vi "RunMeas.vi"(8 "error in (no error)":errorcluster, 11 "ChromaAcLoad in":refnum<class "ChromaAcLoad.lvclass">) -> (0 "error out":errorcluster, 2 "variant":variant, 3 "ChromaAcLoad out":refnum<class "ChromaAcLoad.lvclass">)   [LabVIEW 2018, in "AcPwrPlugins.lvlib" / "ChromaAcLoad.lvclass"]
doc: "This VI (may) initiate the measurement and retrieves the measurement value from the device."
uses:
  ChromaAcLoad.lvclass
  AcPwrShared/clMeasurmentData.ctl
  AcPwrShared/clAcPwrAttributes.ctl
  <instrlib>/C63800/C63800.llb/C63800 M/F Overshoot Voltage.vi
  <instrlib>/C63800/C63800.llb/C63800 M/F Negative Peak Current.vi
  <instrlib>/C63800/C63800.llb/C63800 M/F Undershoot Voltage.vi
  <instrlib>/C63800/C63800.llb/C63800 M/F Apparent Power.vi
  <instrlib>/C63800/C63800.llb/C63800 M/F Power Reactive.vi
  <instrlib>/C63800/C63800.llb/C63800 M/F Power Factor.vi
  AcPwrShared/AcPwrShared.lvlib
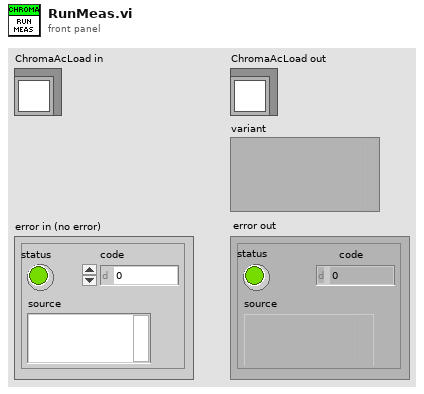
[diagram p1: front panel]
types:
  T1 = typedef "AcPwrPlugins.lvlib/ChromaAcLoad.lvclass/Device(s)Settings.ctl" = cluster{"Configuration Mode":enum16{"Constant Voltage (DC)", "Constant Power (DC)", "Constant Power (AC)", "Constant Current (DC)", "Constant Current (AC)", "Constant Resistance (DC)", "Constant Resistance (AC)", "Rectified Mode (DC)", "Inrush (AC)", "RLC CP (AC)", "RLC (AC)"}, "Phases":cluster{"Handle":string, "Name":string, "Phase Select":i32, "Instrument Options":string, "id query (T)":bool, "reset device (T)":bool, "Load Short Circuited":bool, "Line Synchronization":bool, "Load Current (A/Arms)":dbl, "Load Voltage (V/Vrms)":dbl, "Load Power (W)":dbl, "Load Resistance (Ohms)":dbl, "Load Current Peak Limit (A)":dbl, "Load Current Limit (A/Arms)":dbl, "Load Power Limit (W)":dbl, "Synch Frequency (Hz)":dbl, "Priority":enum16{"CF Only", "PF Only", "Both (CF)", "Both (PF)"}, "Crest Factor":dbl, "Power Factor":dbl, "Slew Rate":cluster{"Rise Slew Rate (A/ms)":i32, "Fall Slew Rate (A/ms)":i32}, "LC/RLC Mode":cluster{"Capacitance (uF)":i32, "Inductance (uH)":i32, "Series Resistance (Ohm)":dbl, "Parallel Resistance (Ohm)":dbl}, "Timing":cluster{"TimingOn":enum16{""}, "Hours":u32, "Minutes":u32, "Seconds":dbl, "CutoffVoltage":dbl}, "Connected":bool}[], "MeasName":string}
  T2 = typedef "AcPwrPlugins.lvlib/ChromaAcLoad.lvclass/Measurements.ctl" = cluster{"Handle":string, "Name":string, "Enabled":bool, "Measurement Value":dbl, "Hold Peak Current Measurement":bool, "btnMeasFetch":bool, "ProtectionStatusString":string, "Measurement Type":T3}[]
  T3 = typedef "AcPwrPlugins.lvlib/ChromaAcLoad.lvclass/MeasurementType.ctl" = enum16{"Voltage (Vrms or V)", "Current (Arms or A)", "Power (W)", "Peak Voltage (V)", "Peak Current (A)", "Peak Power (W)", "Frequency (Hz)", "Resistance (Ohms)", "Voltage Overshoot (V)", "Positive Peak Current (A)", "Voltage Undershoot (V)", "Negative Peak Current (A)", "Apparent Power (VA)", "Reacitive Power (VAR)", "Voltage THD", "Power Factor", "Current's Crest Factor"}
  T4 = typedef "AcPwrShared.lvlib/clMeasurmentData.ctl" = cluster{"MeasName":string, "XML Data":string, "WaveformData":waveform(dbl)[]}
  T5 = typedef "AcPwrShared.lvlib/clAcPwrAttributes.ctl" = cluster{"ProtectionStatusString":string, "Handle_MeasurementType":string, "Status Byte Register":cluster{"Busy":bool, "Remote Mode":bool, "Error in Queue":bool, "QUES=Questionable Status Summary":bool, "MAV = Message Available":bool, "ESB = Event Status Byte Summary":bool, "RQS = Request for Service":bool, "OPER = Operation Event Summary":bool}}
  T6 = cluster{"Handle":string, "Name":string, "Enabled":bool, "Measurement Value":dbl, "Hold Peak Current Measurement":bool, "btnMeasFetch":bool, "ProtectionStatusString":string, "Measurement Type":T3}
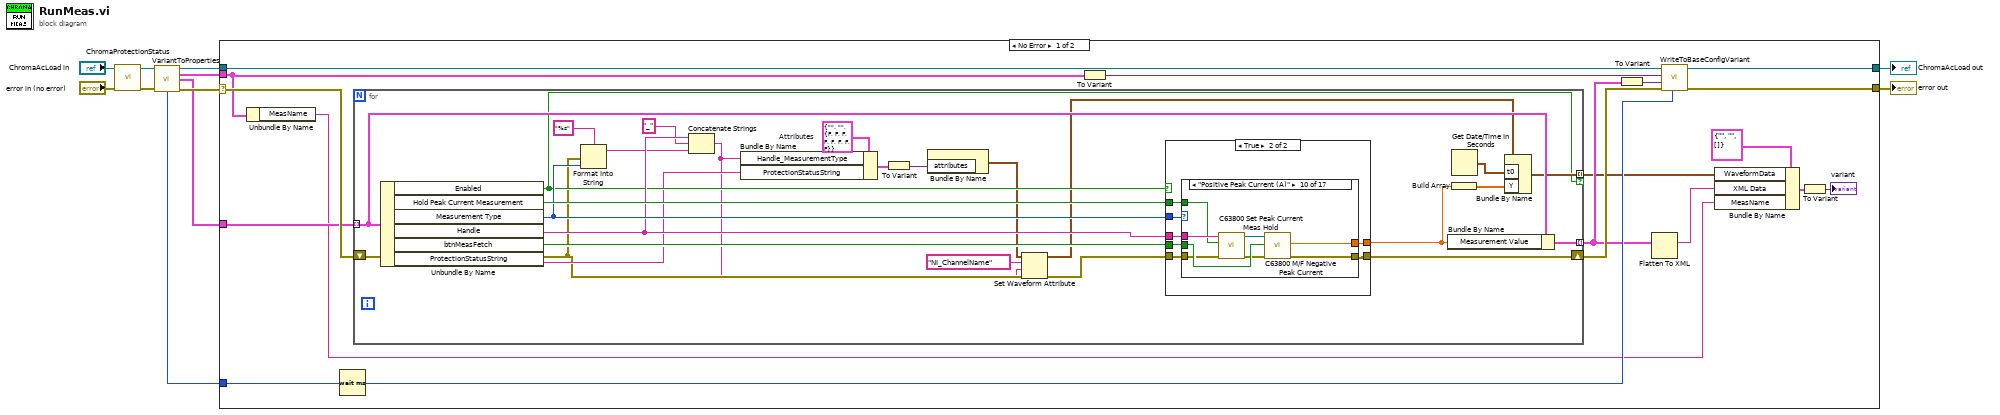
[diagram p0: block diagram]
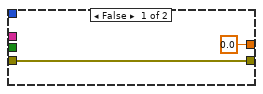
[diagram p2: hidden frame]
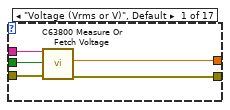
[diagram p3: hidden frame]
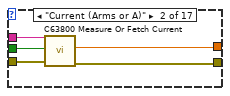
[diagram p4: hidden frame]
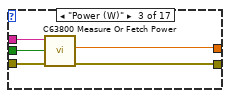
[diagram p5: hidden frame]
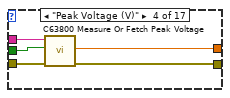
[diagram p6: hidden frame]
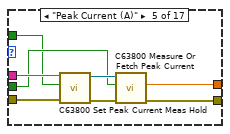
[diagram p7: hidden frame]
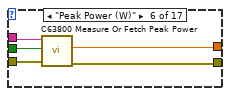
[diagram p8: hidden frame]
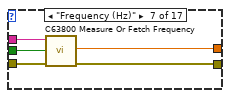
[diagram p9: hidden frame]
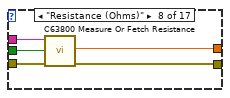
[diagram p10: hidden frame]
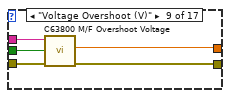
[diagram p11: hidden frame]
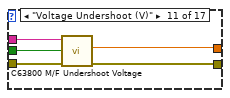
[diagram p12: hidden frame]
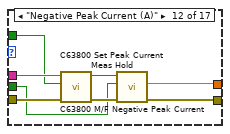
[diagram p13: hidden frame]
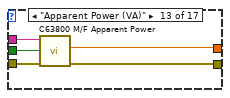
[diagram p14: hidden frame]
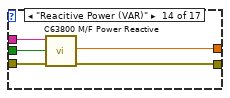
[diagram p15: hidden frame]
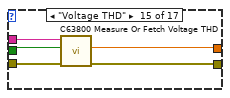
[diagram p16: hidden frame]
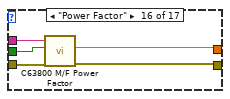
[diagram p17: hidden frame]
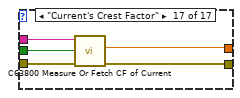
[diagram p18: hidden frame]
diagram:
  n1 = call "ChromaProtectionStatus.vi"("error in (no error)"="error in (no error)", "ChromaAcLoad in"="ChromaAcLoad in") -> ("error out"=w7:errorcluster, "ChromaAcLoad out"=w6:refnum<class "ChromaAcLoad.lvclass">)  [unwired: 8 in]
  n2 = call "VariantToProperties.vi"("ChromaAcLoad"=w6, "error in (no error)"=w7) -> ("ChromaAcLoad"=w5:refnum<class "ChromaAcLoad.lvclass">, "Device Properties"=w2:T1, "Meas"=w3:T2, "Measurement Refresh Time (ms)"=w1:u32, "error out"=w4:errorcluster)  [unwired: 7 in, 2 out]
  n3 = case shown="No Error" w4 {
    selector: w4 -> [w29 w158]
    tunnel: [w25 w159] -> w11
    tunnel: [w23 w158] -> w10
    tunnel: w5 -> [w27 w159]
    tunnel: w2 -> [w20 _]
    tunnel: w3 -> [w28 _]
    tunnel: w1 -> [w21 _]
    frame No Error {
      n4 = Unbundle By Name(w20) -> ("MeasName"=w12:string)
      n5 = Wait (ms)(milliseconds to wait=w21) -> (millisecond timer value=w18:u32)
      n6 = for {
        tunnel: w28 -> [w54] mode=indexing
        shift-right: [w52] -> w26
        shift-left: w29 -> [w32]
        tunnel: [w53] -> w17 mode=indexing
        tunnel: [w47] -> w14 mode=indexing if=w39
        w38 = T5 {"ProtectionStatusString"="", "Handle_MeasurementType"="", "Status Byte Register"={"Busy"=FALSE, "Remote Mode"=FALSE, "Error in Queue"=FALSE, "QUES=Questionable Status Summary"=FALSE, "MAV = Message Available"=FALSE, "ESB = Event Status Byte Summary"=FALSE, "RQS = Request for Service"=FALSE, "OPER = Operation Event Summary"=FALSE}}  # Attributes
        n7 = Unbundle By Name(w54) -> ("Enabled"=w39:bool, "Hold Peak Current Measurement"=w51:bool, "Measurement Type"=w44:T3, "Handle"=w42:string, "btnMeasFetch"=w50:bool, "ProtectionStatusString"=w36:string)
        n8 = Format Into String(format string="%s", error in=w32, w44) -> (resulting string=w40:string)  [unwired: 1 in, 1 out]
        n9 = Concatenate Strings(w42, "_", w40) -> (w31:string)
        n10 = Bundle By Name(cluster=w38, "Handle_MeasurementType"=w31, "ProtectionStatusString"=w36) -> (w37:T5)
        n11 = To Variant(anything=w37) -> (Variant=w43:variant)
        n12 = Bundle By Name("attributes"=w43) -> (w30:waveform(dbl))  [unwired: 1 in]
        n13 = Set Waveform Attribute(4:w32, 5:w31, 6:"NI_ChannelName" ("name"), 7:w30) -> (0:w34:errorcluster, 3:w33:waveform(dbl))  [unwired: 1 out]
        n14 = case shown="True" w39 {
          tunnel: w34 -> [w56 w63]
          tunnel: w44 -> [_ w60]
          tunnel: [w56 w58] -> w52
          tunnel: [0.0 ("Query CF of Current") w57] -> w49
          tunnel: w42 -> [_ w62]
          tunnel: w51 -> [_ w59]
          tunnel: w50 -> [_ w61]
          frame False {
          }
          frame True {
            n15 = case shown="\"Positive Peak Current (A)\"" w60 {
              tunnel: w63 -> [w68 w71 w76 w83 w87 w94 w101 w106 w111 w114 w124 w128 w137 w142 w147 w152 w156]
              tunnel: w62 -> [w67 w70 w74 w81 w86 w92 w98 w102 w107 w113 w123 w127 w136 w138 w145 w151 w155]
              tunnel: w61 -> [w66 w69 w75 w82 w85 w93 w97 w103 w108 w117 w122 w126 w135 w139 w144 w150 w154]
              tunnel: w59 -> [_ _ _ _ w84 _ _ _ _ w112 _ w125 _ _ _ _ _]
              tunnel: [w65 w73 w78 w80 w91 w96 w100 w105 w110 w119 w121 w132 w134 w141 w146 w149 w157] -> w58
              tunnel: [w64 w72 w77 w79 w90 w95 w99 w104 w109 w118 w120 w131 w133 w140 w143 w148 w153] -> w57
              frame "Voltage (Vrms or V)", Default {
                n16 = call <instrlib>:"C63800 Measure Or Fetch Voltage.vi"("error in (no error)"=w68, "Query Type"=w66, "Instrument Handle"=w67) -> ("error out"=w65:errorcluster, "Query Voltage"=w64:dbl)  [unwired: 6 in, 1 out]
              }
              frame "Current (Arms or A)" {
                n17 = call <instrlib>:"C63800 Measure Or Fetch Current.vi"("error in (no error)"=w71, "Query Type"=w69, "Instrument Handle"=w70) -> ("error out"=w73:errorcluster, "Query Current"=w72:dbl)  [unwired: 6 in, 1 out]
              }
              frame "Power (W)" {
                n18 = call <instrlib>:"C63800 Measure Or Fetch Power.vi"("error in (no error)"=w76, "Query Type"=w75, "Instrument Handle"=w74) -> ("error out"=w78:errorcluster, "Query Power"=w77:dbl)  [unwired: 6 in, 1 out]
              }
              frame "Peak Voltage (V)" {
                n19 = call <instrlib>:"C63800 Measure Or Fetch Peak Voltage.vi"("error in (no error)"=w83, "Query Type"=w82, "Instrument Handle"=w81) -> ("error out"=w80:errorcluster, "Query Peak Voltage"=w79:dbl)  [unwired: 6 in, 1 out]
              }
              frame "Peak Current (A)" {
                n20 = call <instrlib>:"C63800 Set Peak Current Meas Hold.vi"("error in (no error)"=w87, "Hold State"=w84, "Instrument Handle"=w86) -> ("error out"=w89:errorcluster, "Instrument Handle out"=w88:refnum<k15>)  [unwired: 7 in]
                n21 = call <instrlib>:"C63800 Measure Or Fetch Peak Current.vi"("error in (no error)"=w89, "Query Type"=w85, "Instrument Handle"=w88) -> ("error out"=w91:errorcluster, "Query Peak Current"=w90:dbl)  [unwired: 6 in, 1 out]
              }
              frame "Peak Power (W)" {
                n22 = call <instrlib>:"C63800 Measure Or Fetch Peak Power.vi"("error in (no error)"=w94, "Query Type"=w93, "Instrument Handle"=w92) -> ("error out"=w96:errorcluster, "Query Peak Power"=w95:dbl)  [unwired: 6 in, 1 out]
              }
              frame "Frequency (Hz)" {
                n23 = call <instrlib>:"C63800 Measure Or Fetch Frequency.vi"("error in (no error)"=w101, "Query Type"=w97, "Instrument Handle"=w98) -> ("error out"=w100:errorcluster, "Query Frequency"=w99:dbl)  [unwired: 6 in, 1 out]
              }
              frame "Resistance (Ohms)" {
                n24 = call <instrlib>:"C63800 Measure Or Fetch Resistance.vi"("error in (no error)"=w106, "Query Type"=w103, "Instrument Handle"=w102) -> ("error out"=w105:errorcluster, "Query Resistance"=w104:dbl)  [unwired: 6 in, 1 out]
              }
              frame "Voltage Overshoot (V)" {
                n25 = call "C63800 M/F Overshoot Voltage.vi"("error in (no error)"=w111, "Query Type"=w108, "Instrument Handle"=w107) -> ("error out"=w110:errorcluster, "Query Overshoot Voltage"=w109:dbl)  [unwired: 6 in, 1 out]
              }
              frame "Positive Peak Current (A)" {
                n26 = call <instrlib>:"C63800 Set Peak Current Meas Hold.vi"("error in (no error)"=w114, "Hold State"=w112, "Instrument Handle"=w113) -> ("error out"=w116:errorcluster, "Instrument Handle out"=w115:refnum<k15>)  [unwired: 7 in]
                n27 = call "C63800 M/F Negative Peak Current.vi"("error in (no error)"=w116, "Query Type"=w117, "Instrument Handle"=w115) -> ("error out"=w119:errorcluster, "Query Negative Peak Current"=w118:dbl)  [unwired: 6 in, 1 out]
              }
              frame "Voltage Undershoot (V)" {
                n28 = call "C63800 M/F Undershoot Voltage.vi"("error in (no error)"=w124, "Query Type"=w122, "Instrument Handle"=w123) -> ("error out"=w121:errorcluster, "Query Undershoot Voltage"=w120:dbl)  [unwired: 6 in, 1 out]
              }
              frame "Negative Peak Current (A)" {
                n29 = call <instrlib>:"C63800 Set Peak Current Meas Hold.vi"("error in (no error)"=w128, "Hold State"=w125, "Instrument Handle"=w127) -> ("error out"=w130:errorcluster, "Instrument Handle out"=w129:refnum<k15>)  [unwired: 7 in]
                n30 = call "C63800 M/F Negative Peak Current.vi"("error in (no error)"=w130, "Query Type"=w126, "Instrument Handle"=w129) -> ("error out"=w132:errorcluster, "Query Negative Peak Current"=w131:dbl)  [unwired: 6 in, 1 out]
              }
              frame "Apparent Power (VA)" {
                n31 = call "C63800 M/F Apparent Power.vi"("error in (no error)"=w137, "Query Type"=w135, "Instrument Handle"=w136) -> ("error out"=w134:errorcluster, "Query Apparent Power"=w133:dbl)  [unwired: 6 in, 1 out]
              }
              frame "Reacitive Power (VAR)" {
                n32 = call "C63800 M/F Power Reactive.vi"("error in (no error)"=w142, "Query Type"=w139, "Instrument Handle"=w138) -> ("error out"=w141:errorcluster, "Query Power Reactive"=w140:dbl)  [unwired: 6 in, 1 out]
              }
              frame "Voltage THD" {
                n33 = call <instrlib>:"C63800 Measure Or Fetch Voltage THD.vi"("error in (no error)"=w147, "Query Type"=w144, "Instrument Handle"=w145) -> ("error out"=w146:errorcluster, "Query Voltage THD"=w143:dbl)  [unwired: 6 in, 1 out]
              }
              frame "Power Factor" {
                n34 = call "C63800 M/F Power Factor.vi"("error in (no error)"=w152, "Query Type"=w150, "Instrument Handle"=w151) -> ("error out"=w149:errorcluster, "Query PF"=w148:dbl)  [unwired: 6 in, 1 out]
              }
              frame "Current's Crest Factor" {
                n35 = call <instrlib>:"C63800 Measure Or Fetch CF of Current.vi"("error in (no error)"=w156, "Query Type"=w154, "Instrument Handle"=w155) -> ("error out"=w157:errorcluster, "Query CF of Current"=w153:dbl)  [unwired: 6 in, 1 out]
              }
            }
          }
        }
        n36 = Bundle By Name(cluster=w54, "Measurement Value"=w49) -> (w53:T6)
        n37 = Build Array(w49) -> (w48:dbl[])
        n38 = Get Date/Time In Seconds() -> (seconds since 1Jan1904=w46:timestamp)
        n39 = Bundle By Name(cluster=w33, "t0"=w46, "Y"=w48) -> (w47:waveform(dbl))
      }
      n40 = To Variant(anything=w20) -> (Variant=w22:variant)
      n41 = To Variant(anything=w17) -> (Variant=w24:variant)
      n42 = Flatten To XML(anything=w17) -> (xml string=w13:string)
      n43 = call "WriteToBaseConfigVariant.vi"("Measurement Refresh Time (ms)"=w18, "error in (no error)"=w26, "Meas"=w24, "Config"=w22, "ChromaAcLoad in"=w27) -> ("error out"=w23:errorcluster, "ChromaAcLoad out"=w25:refnum<class "ChromaAcLoad.lvclass">)  [unwired: 5 in]
      n44 = Bundle By Name(cluster=T4 {"MeasName"="", "XML Data"="", "WaveformData"=[]} ("MeasurmentDataCluster"), "WaveformData"=w14, "XML Data"=w13, "MeasName"=w12) -> (w15:T4)
      n45 = To Variant(anything=w15) -> (Variant=→"variant":variant)
    }
    frame Error {
    }
  }
  "ChromaAcLoad out" <- w11
  "error out" <- w10
